vi "MT Map Bits to ASK Symbols.vi"(0 "input bit stream":i8[](array[numeric]), 5 "symbol map":cdb[](array[numeric]) format="%.3f", 11 "error in (no error)":errorcluster, 13 "reset? (T)":bool=TRUE) -> (4 "symbols":cdb[](array[numeric]) format="%.3f", 15 "error out":errorcluster)   [LabVIEW 2020, in "niDMT.lvlib"]
doc: "This polymorphic instance maps an incoming bit stream to complex-valued ASK symbols."
uses:
  <vilib>/addons/Modulation/niDMT.lvlib
  <vilib>/addons/Modulation/niAMT.lvlib
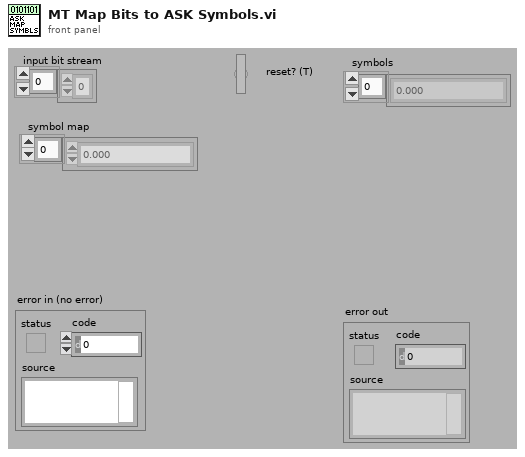
[diagram p1: front panel]
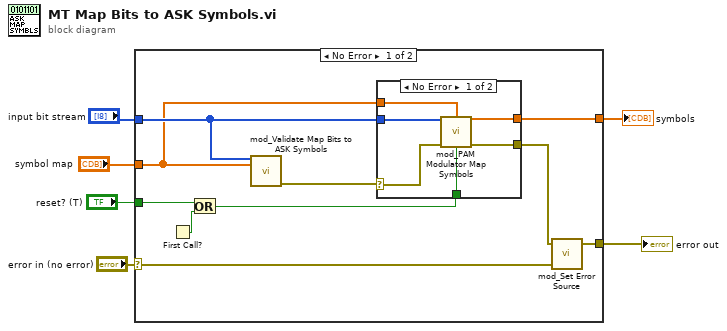
[diagram p0: block diagram]
diagram:
  n1 = case shown="No Error" "error in (no error)" {
    selector: "error in (no error)" -> [w8 w24]
    tunnel: "reset? (T)" -> [w16 _]
    tunnel: "input bit stream" -> [w12 _]
    tunnel: [w13 _] -> w3
    tunnel: [w10 w24] -> w2
    tunnel: "symbol map" -> [w7 _]
    frame No Error {
      n2 = First Call?() -> (First Call?: T/F=w15:bool)
      n3 = Or(x=w16, y=w15) -> (x .or. y?=w14:bool)
      n4 = call <vilib>:"mod_Validate Map Bits to ASK Symbols.vi"("input bit stream"=w12, "symbol map"=w7) -> ("error out"=w11:errorcluster)  [unwired: 13 out]
      n5 = case shown="No Error" w11 {
        selector: w11 -> [w18 w23]
        tunnel: w14 -> [w22 _]
        tunnel: [w21 _] -> w13
        tunnel: [w20 w23] -> w9
        tunnel: w12 -> [w19 _]
        tunnel: w7 -> [w17 _]
        frame No Error {
          n6 = call <vilib>:"mod_PAM Modulator Map Symbols.vi"("Input Bit Stream"=w19, "Symbol Map"=w17, "error in (no error)"=w18, "Reset? (T)"=w22) -> ("Symbols"=w21:cdb[], "error out"=w20:errorcluster)  [unwired: 1 in, 9 out]
        }
        frame Error {
        }
      }
      n7 = call <vilib>:"mod_Set Error Source.vi"("initial error in (no error)"=w8, "final error in (no error)"=w9) -> ("error out"=w10:errorcluster)  [unwired: 3 out]
    }
    frame Error {
    }
  }
  "symbols" <- w3
  "error out" <- w2
